vi "Get SMO Public API.vi"(8 "error in (no error)":errorcluster, 11 "Instrument.TC in":refnum<class "Instrument.TC.lvclass">) -> (0 "error out":errorcluster, 2 "Commands":string[](array[string]), 3 "Instrument.TC out":refnum<class "Instrument.TC.lvclass">)   [LabVIEW 2019, in "Instrument.TC.lvclass"]
uses:
  Instrument.TC.lvclass
  <userlib>/LevyLab/Instrument Framework/Instrument Types/Cryostat/Instrument.Cryostat.lvclass
  Typedefs/Commands--enum.ctl
  <userlib>/LevyLab/Instrument Framework/SMOs/Instrument/Instrument.lvclass
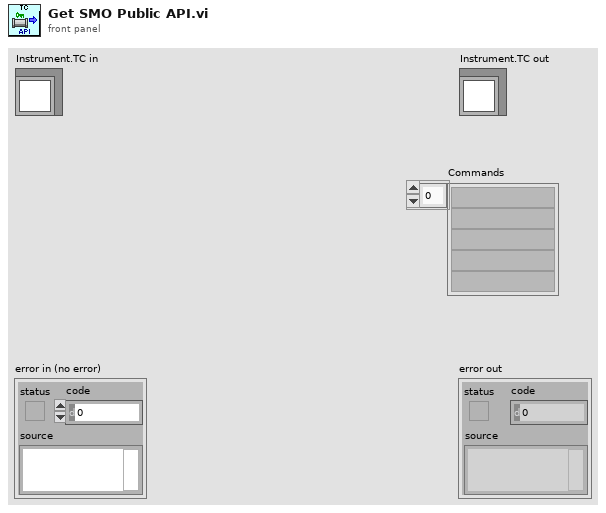
[diagram p1: front panel]
types:
  T1 = typedef "Instrument.TC.lvclass/Commands--enum.ctl" = enum16{"Set Heater"}
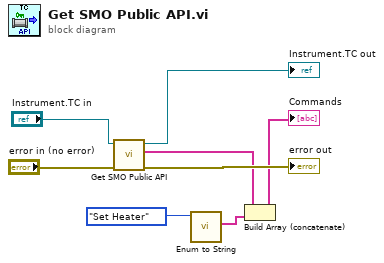
[diagram p0: block diagram]
diagram:
  n1 = call-parent "Get SMO Public API.vi"("error in (no error)"="error in (no error)", "Instrument in"="Instrument.TC in") -> ("error out"=→"error out":errorcluster, "Commands"=w2:string[], "Instrument out"=→"Instrument.TC out":refnum<class "Instrument.TC.lvclass">)  [unwired: 7 in]
  n2 = call <userlib>:"Enum to String.vi"("Command"=Commands--enum."Set Heater") -> ("Commands []"=w3:string[])  [unwired: 9 in, 1 out]
  n3 = Build Array (concatenate)(w2, w3) -> (→"Commands":string[])
